vi "LVClass_HasoData Get DimensionsAndSteps.vi"(0 "HasoData in":refnum<class "HasoData.lvclass">, 11 "error in (no error)":errorcluster) -> (4 "HasoData out":refnum<class "HasoData.lvclass">, 8 "Dimensions":cluster{"size":T1, "steps":T2}, 15 "error out":errorcluster)   [LabVIEW 2020, in "HasoData.lvclass"]
doc: "Get HasoData dimensions and steps.\n\n--------------------------------------------------------------------------------\n\n<B>HasoDataIn </B> : HasoData object.\n<B>HasoDataOut </B> : HasoData object.\n<B>dimensions </B> : HasoData dimensions as the (width, height) of the pupil.\n<B>steps </B> : HasoData sampling steps in x and y direction (um).\n<B>ErrorIn </B> : Error\n<B>ErrorOut </B> : Error\n\n--------------------------------------------------------------------------------"
uses:
  HasoData.lvclass
  Point2D.ctl
  Point2Df.ctl
  HasoData.lvclass/HasoData.ctl
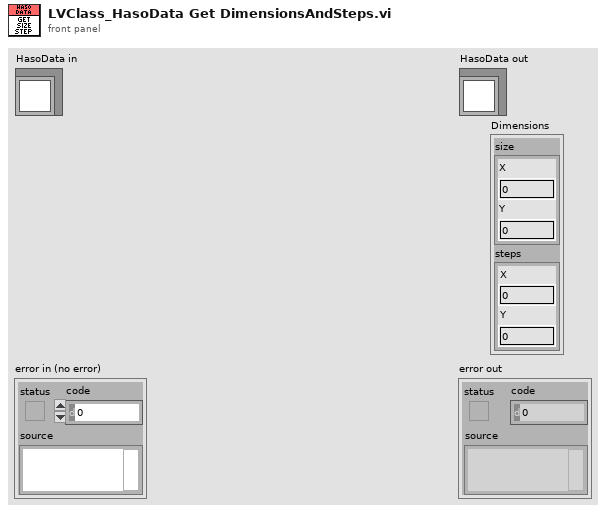
[diagram p1: front panel]
types:
  T1 = typedef "Point2D.ctl" = cluster{"X":u32, "Y":u32}
  T2 = typedef "Point2Df.ctl" = cluster{"X":sgl, "Y":sgl}
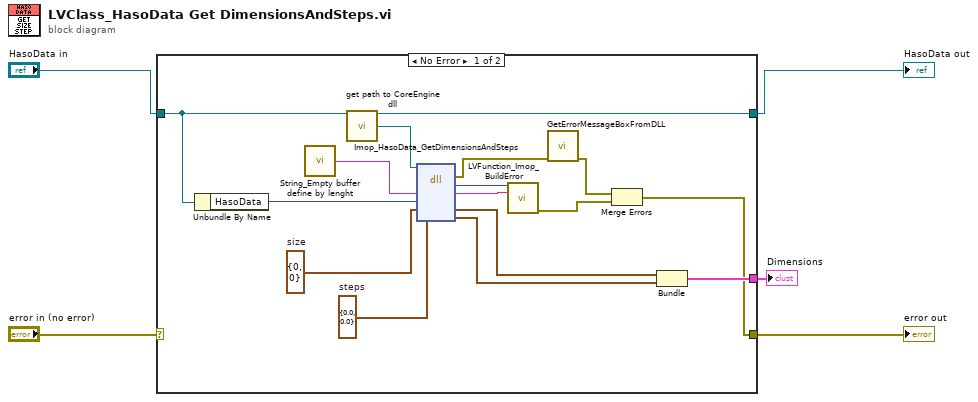
[diagram p0: block diagram]
diagram:
  n1 = case shown="No Error" "error in (no error)" {
    selector: "error in (no error)" -> [_ w22]
    tunnel: [w6 w22] -> w3
    tunnel: [w13 w21] -> w2
    tunnel: "HasoData in" -> [w13 w21]
    tunnel: [w10 _] -> w1
    frame No Error {
      w14 = T2 {"X"=0.0, "Y"=0.0}  # steps
      w15 = T1 {"X"=0, "Y"=0}  # size
      n2 = Unbundle By Name(w13) -> ("HasoData"=w12:i32)
      n3 = call "String_Empty buffer define by lenght.vi"() -> ("Empty buffer"=w18:string)  [unwired: 1 in]
      n4 = call "get path to CoreEngine dll.vi"() -> ("path to c_interface_vc100.dll"=w17:path)  [unwired: 12 in, 3 out]
      n5 = dll-call lib="D:/soft/HASO_v3/SVN_trunk/ImOpCoreEngine4_LV2011/DLLs/c_interface_vc100.dll" fn="Imop_HasoData_GetDimensionsAndSteps"(path in=w17, "message"=w18, "HasoData"=w12, "size"=w15, "steps"=w14) -> (error out=w16:errorcluster, "return type"=w20:i32, "message"=w19:string, "size"=w11:T1, "steps"=w9:T2)  [unwired: 3 in, 1 out]
      n6 = call "LVFunction_Imop_BuildError.vi"("code"=w20, "String to Prepend to source (\"\")"=w19) -> ("error out"=w7:errorcluster)  [unwired: 13 in]
      n7 = call "GetErrorMessageBoxFromDLL.vi"("error IN"=w16) -> ("error OUT"=w8:errorcluster)  [unwired: 10 in]
      n8 = Merge Errors(w8, w7) -> (w6:errorcluster)
      n9 = Bundle("size"=w11, "steps"=w9) -> (w10:cluster{"size":T1, "steps":T2})  [unwired: 1 in]
    }
    frame Error {
    }
  }
  "error out" <- w3
  "HasoData out" <- w2
  "Dimensions" <- w1
